vi "emballage nouvelle série_GPAO_OLD.vi"(1 "CodeBarFix":string, 2 "Nom du produit":string="12-216E-01-25 F120023 500mA 10Ohm", 3 "error in (no error)":errorcluster caption="entrée d'erreur (pas d'erreur)", 6 "Verif.Indice Client":bool) -> (5 "error out":errorcluster caption="sortie d'erreur", 11 "Indice Client":string, 14 "No commande FAS":string, 16 "DATA cmde":T1={"n°article FAS"="12-216E-01-25 F120023 500mA 10ohm", "n° cmde FAS"="R03844/08-01.01.01", "quantité cmde"="4", "ID LIG cmde"="225540", "n° cmde client"="120565              ", "nom client"="Fluid Automat. Systems GmbH", "n° article client"="21088", "indice revision client"="      ", "société de facturation"="FAS Medic SA                            ", "langue a utiliser"="ALL"}, 17 "Quantité de la commande":string="4", 18 "Commande interne":bool, 19 "Annuler(T=OK)":bool)   [LabVIEW 2020]
uses:
  VG_VerifTests_ModeRetour.vi
  Modules/FS/60_FS_Controles/60_FS_SetGet.ctl
panel:
  out "Cde_GPAO":bool
  in  "Cmde_Interne?":bool
  out "Indice Piece":string
  out "Tableau historique":string[][](array[string])=[["112105740008090004", "01.01.2001 01:01:00", "55", "01234/08-01.01.01", "1", "0"], ["112105740008090006", "01.01.2001 01:01:00", "55", "56789/08-01.01.01", "3", "0"], ["112105740008090007", "01.01.2001 01:01:00", "55", "56789/08-01.01.01", "4", "0"], ["112105740008090007", "01.01.2001 01:01:00", "55", "00123/08-01.01.01", "2", "1"]]
  out "Glissière 2":u8(slide)=100 caption="Identification terminé." scale=0.0..100.0
  in  "Valider qtté":bool
  in  "modifier qtté":bool
  in  "Numéro de commande FAS":string(combo)
  in  "Valider cmde":bool
  in  "Annuler?":bool
  # "La recherche se fait uniquement avec le numéro d'article et du numéro de file.\nLa designation (24V,...) n'est pas tenue compte (sauf pour les Flatprop) !!"
  # "Numéro de commande FAS"
  # "Seul un responsable peut valider une commande R (Retour)"
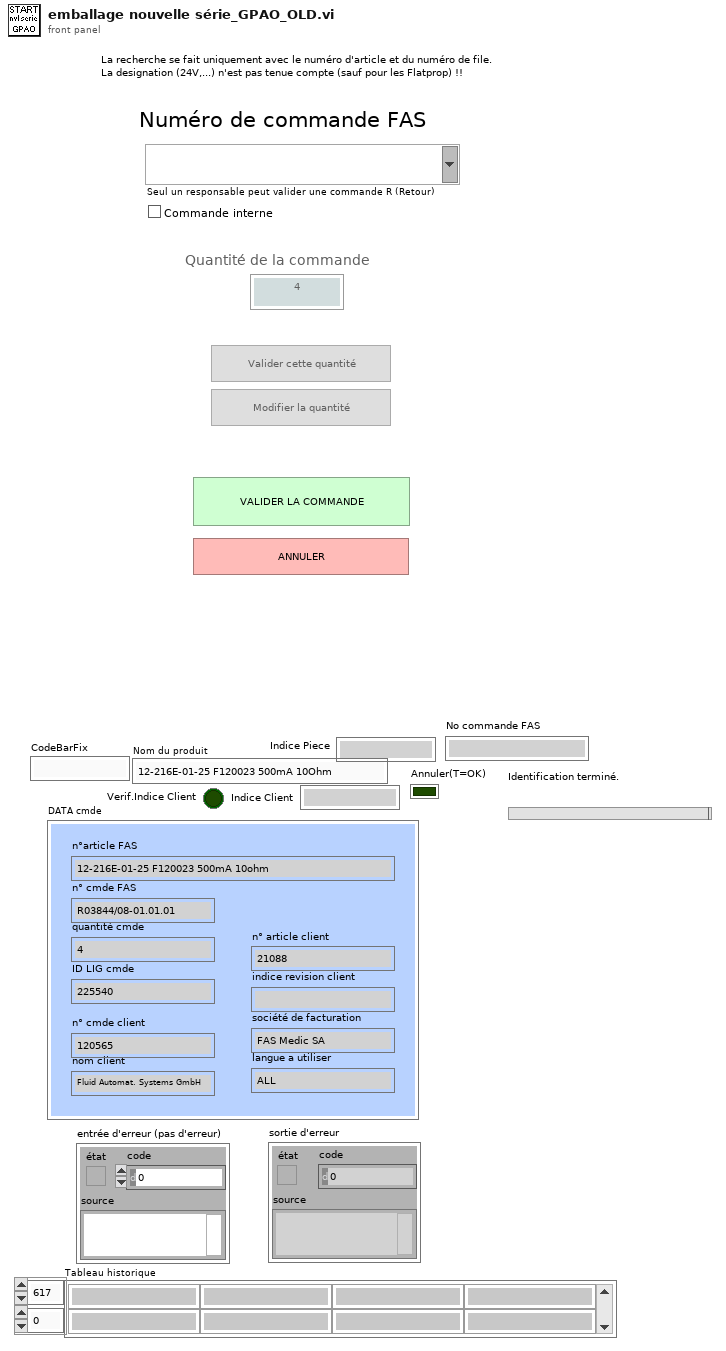
[diagram p1: front panel]
types:
  T1 = typedef "DATA commande.ctl" = cluster{"n°article FAS":string, "n° cmde FAS":string, "quantité cmde":string, "ID LIG cmde":string, "n° cmde client":string, "nom client":string, "n° article client":string, "indice revision client":string, "société de facturation":string, "langue a utiliser":string}
  T2 = typedef "60_FS_SetGet.ctl" = enum16{"set", "get"}
  T3 = enum16{"n° produit", "date", "opérateur", "n° cmde", "n° carton"}
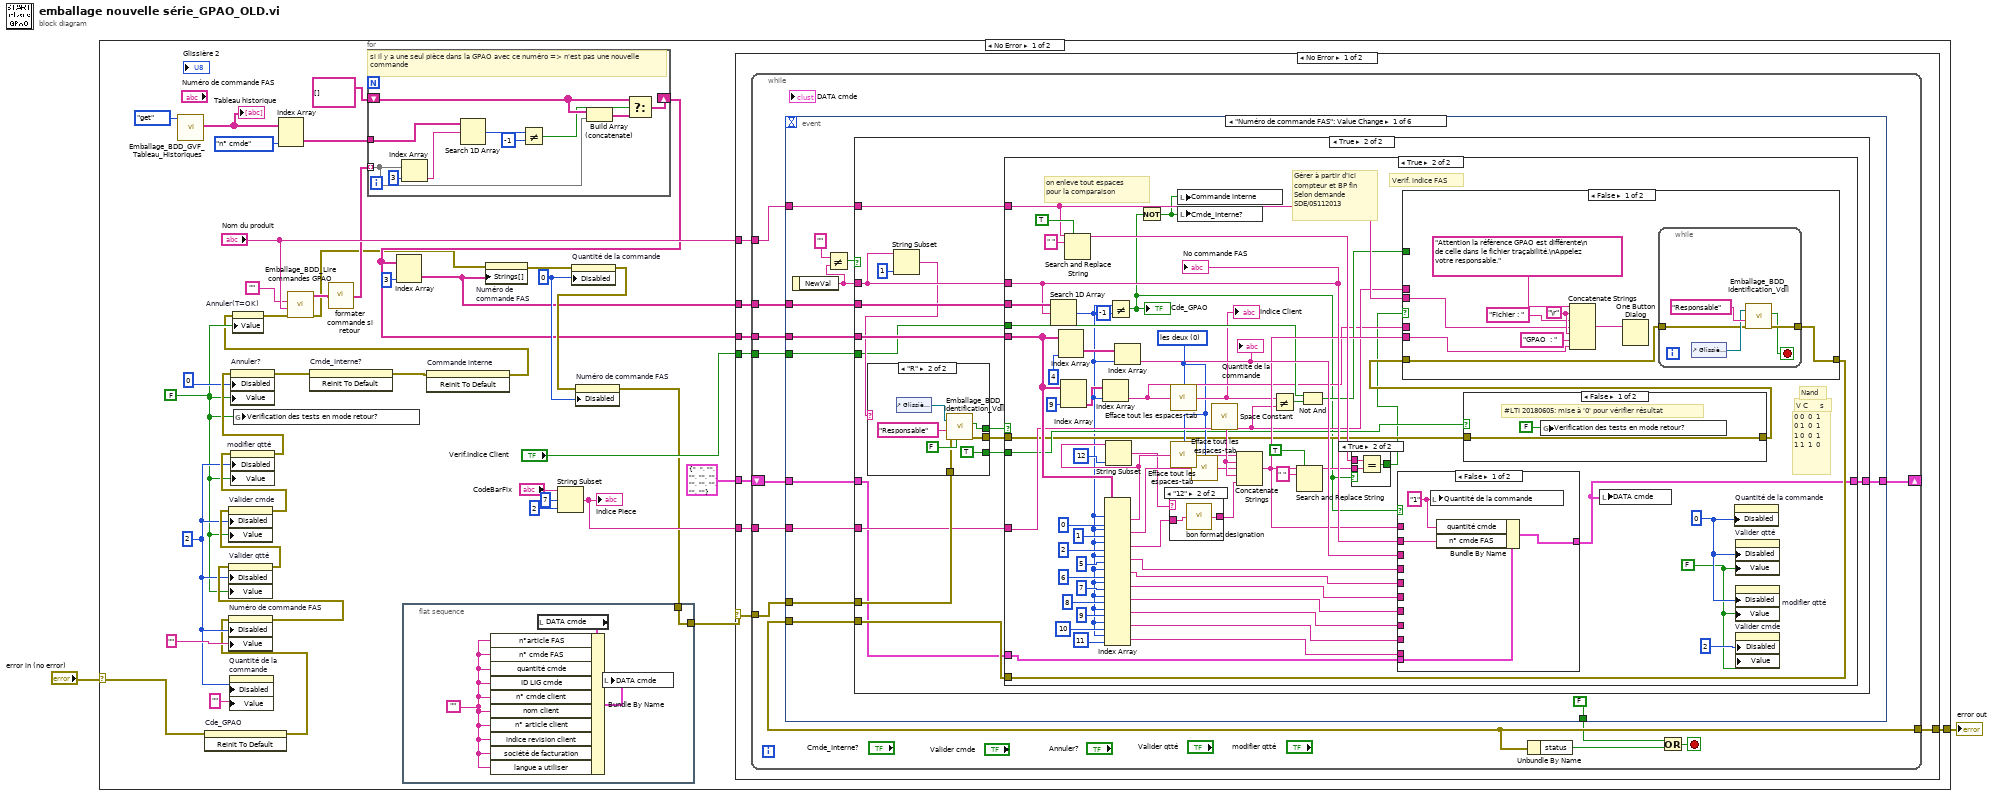
[diagram p0: block diagram]
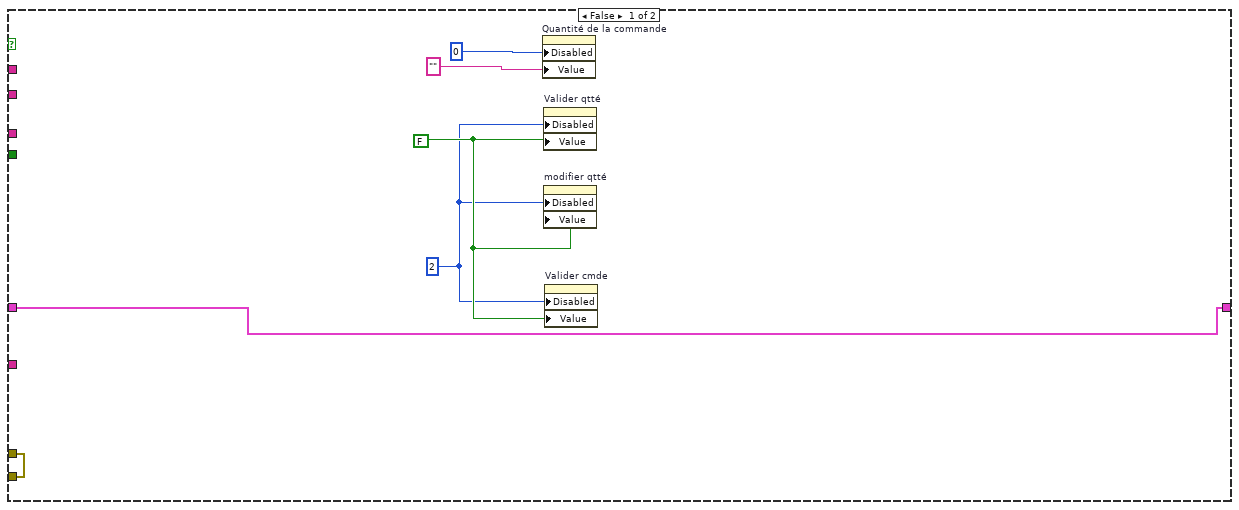
[diagram p2: hidden frame]
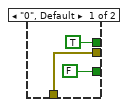
[diagram p3: hidden frame]
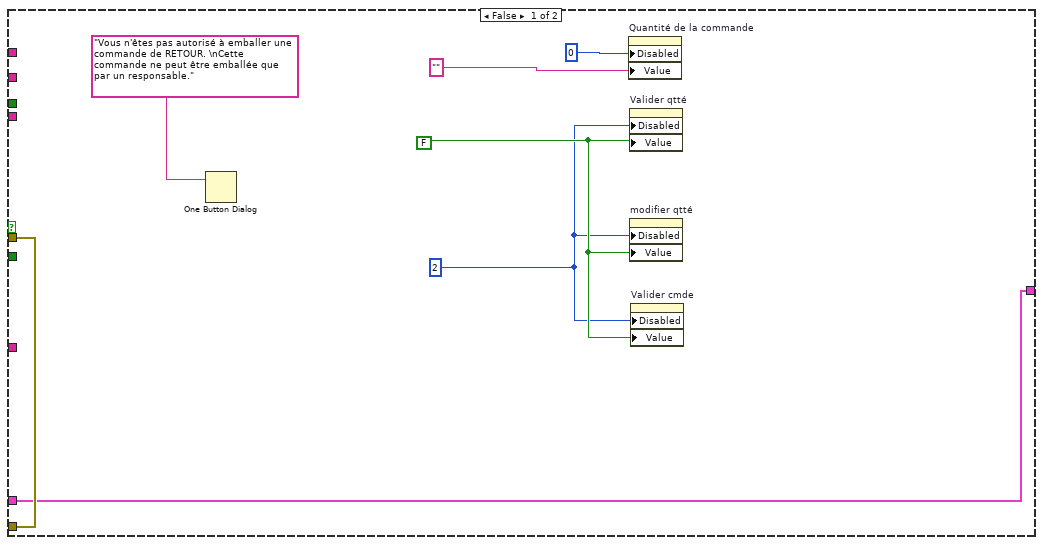
[diagram p4: hidden frame]
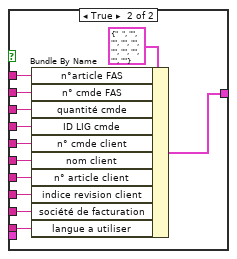
[diagram p5: hidden frame]
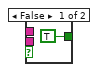
[diagram p6: hidden frame]
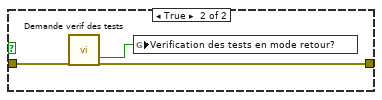
[diagram p7: hidden frame]
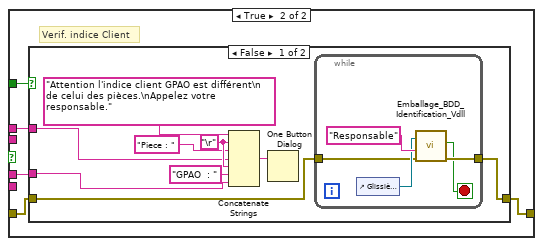
[diagram p8: hidden frame]
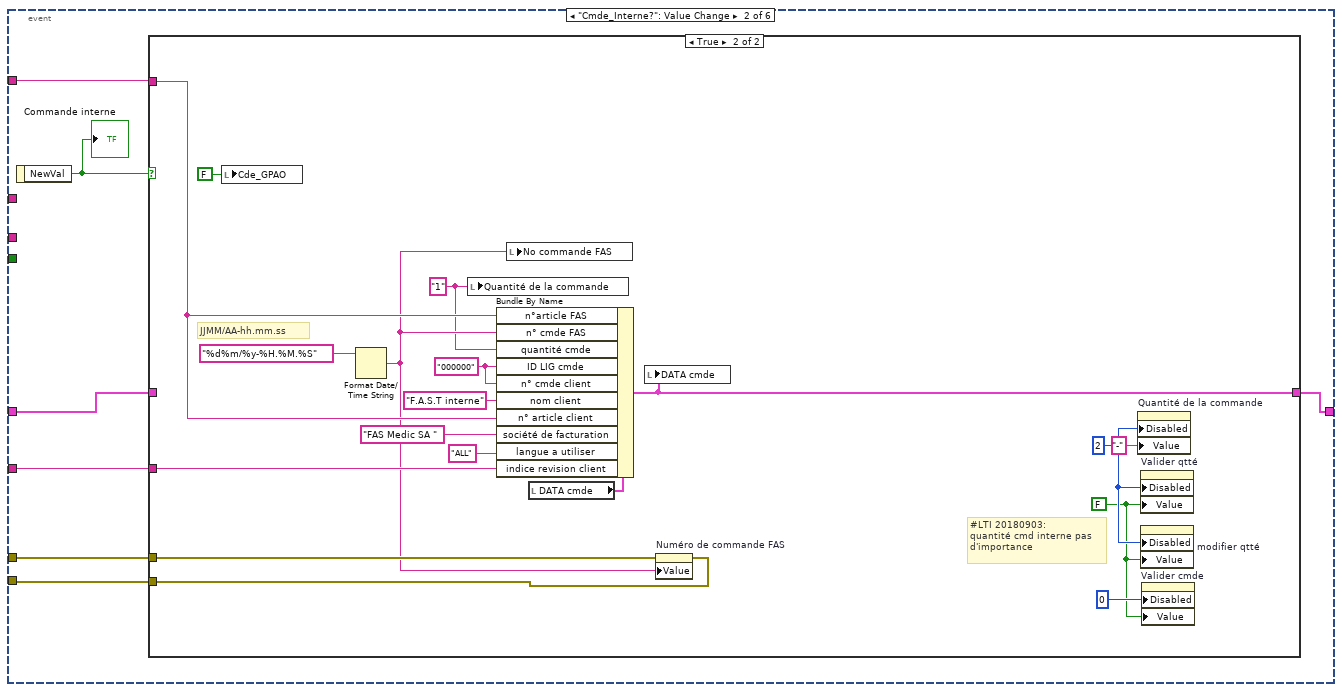
[diagram p11: hidden frame]
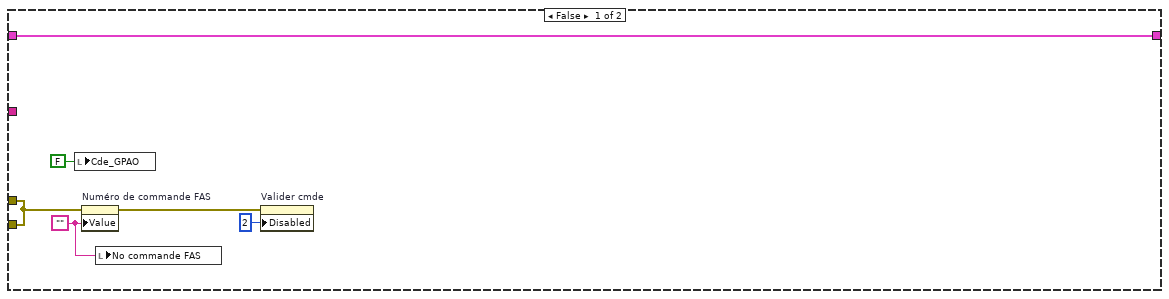
[diagram p12: hidden frame]
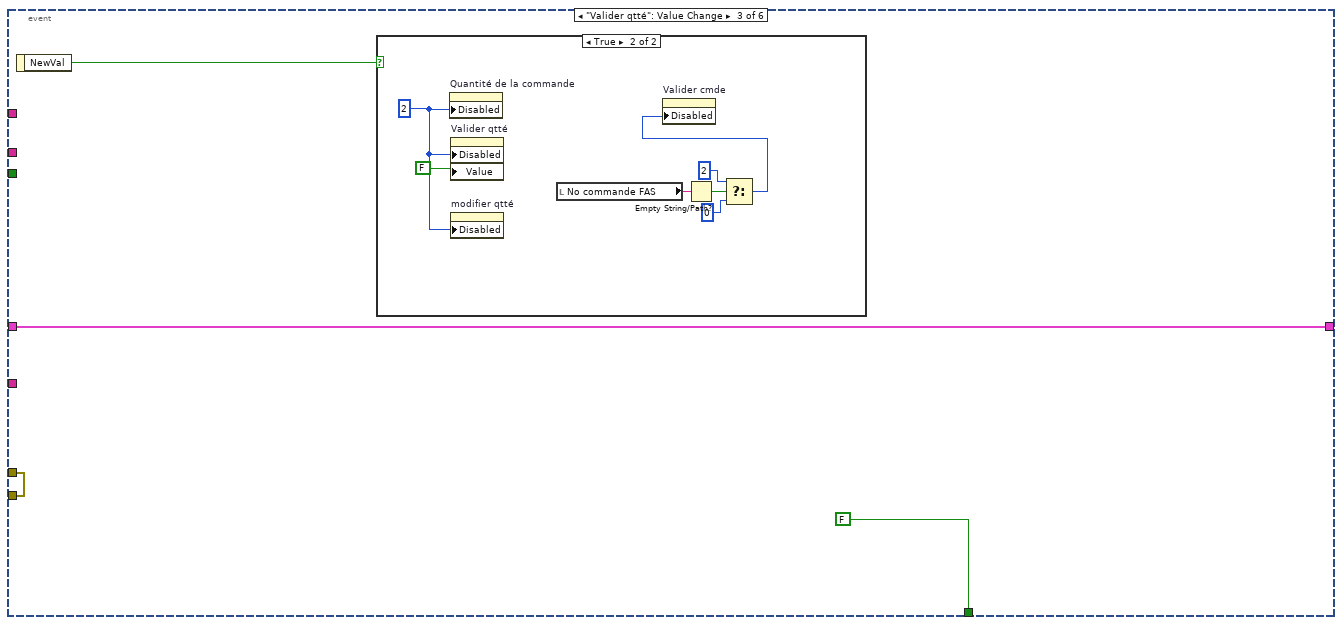
[diagram p13: hidden frame]
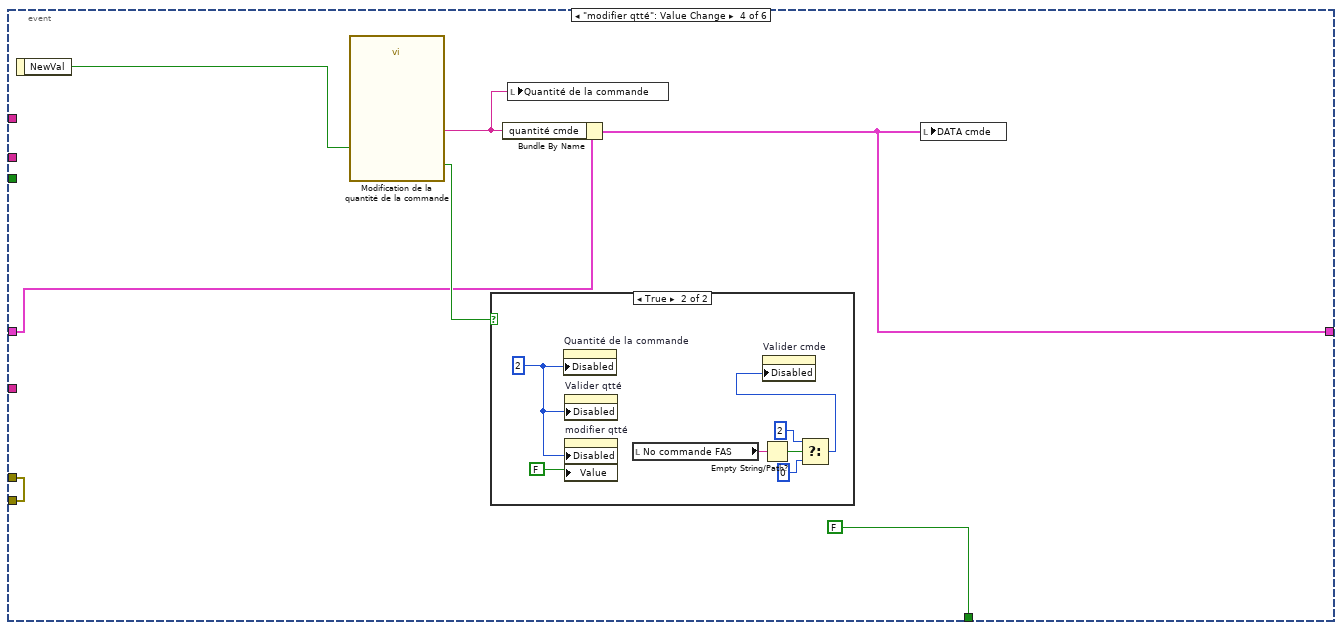
[diagram p15: hidden frame]
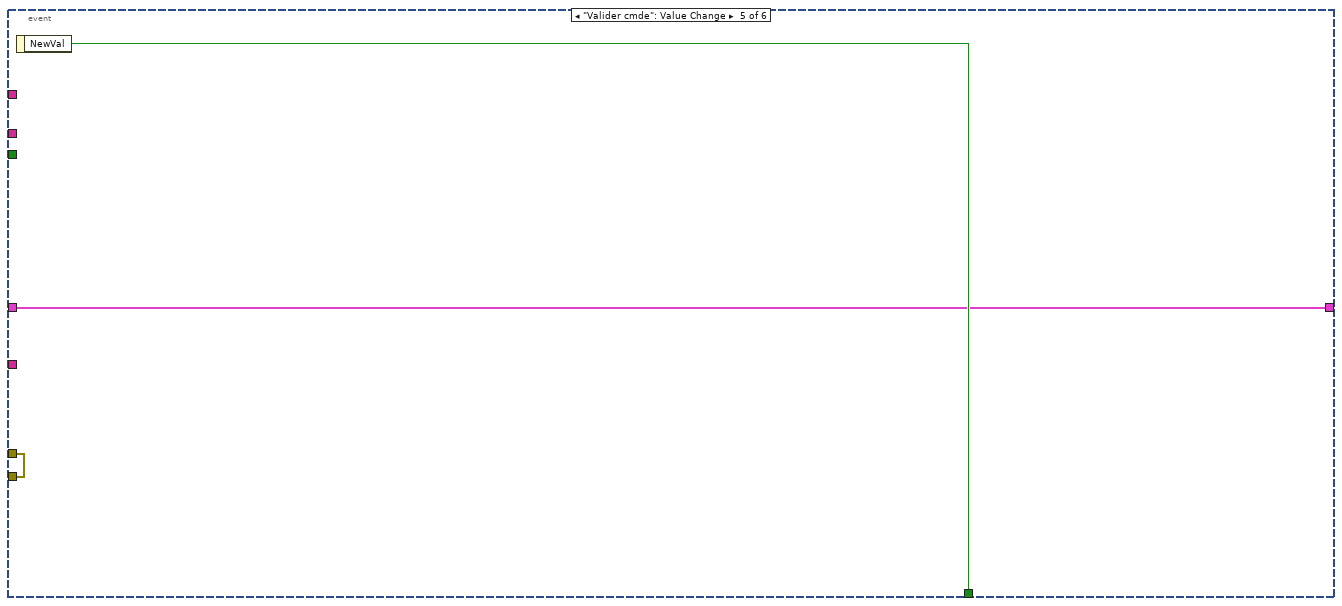
[diagram p17: hidden frame]
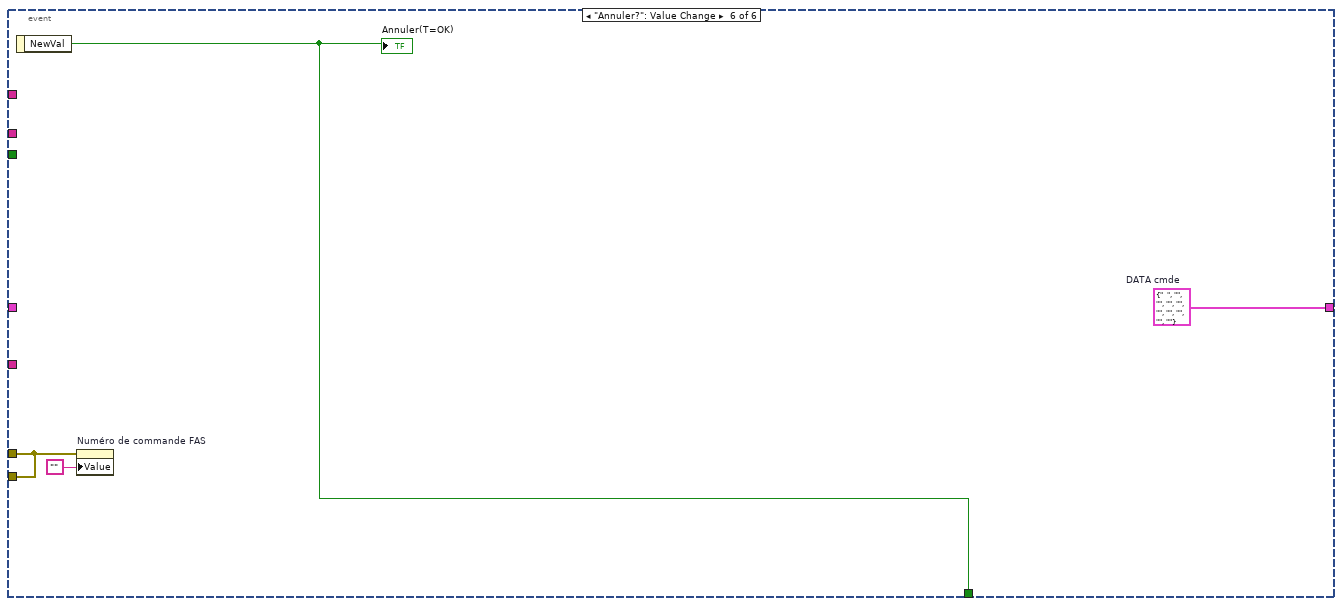
[diagram p18: hidden frame]
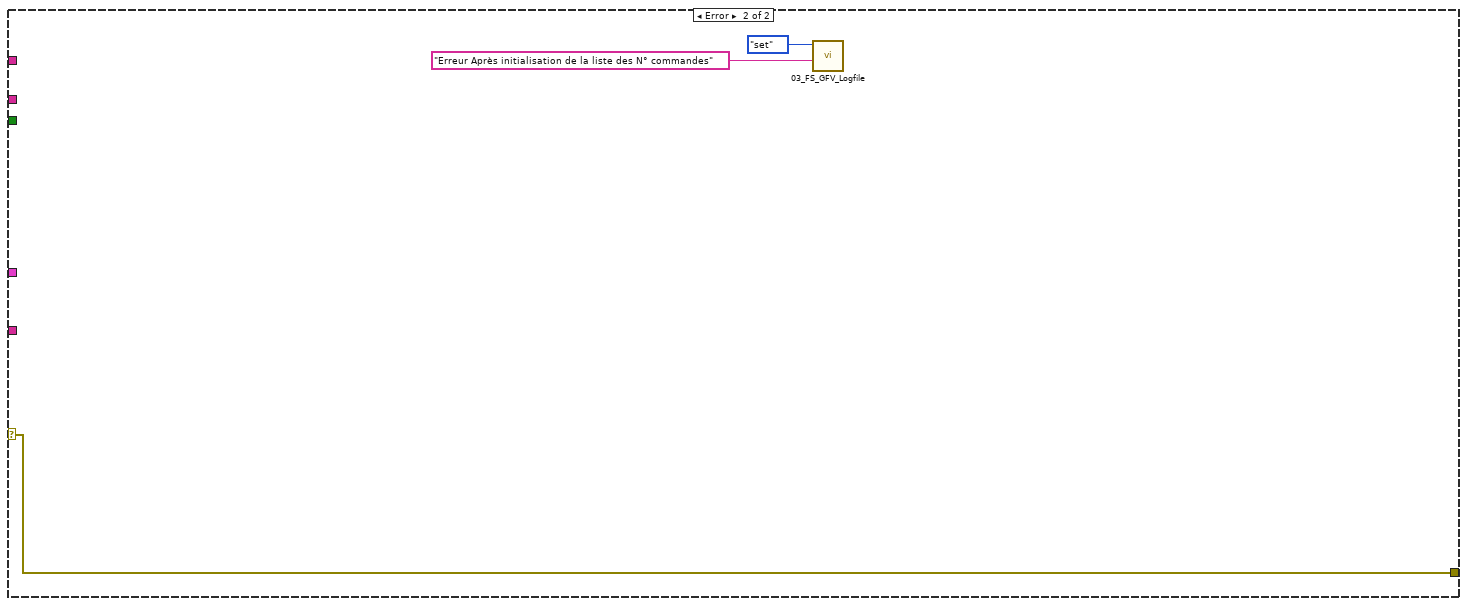
[diagram p19: hidden frame]
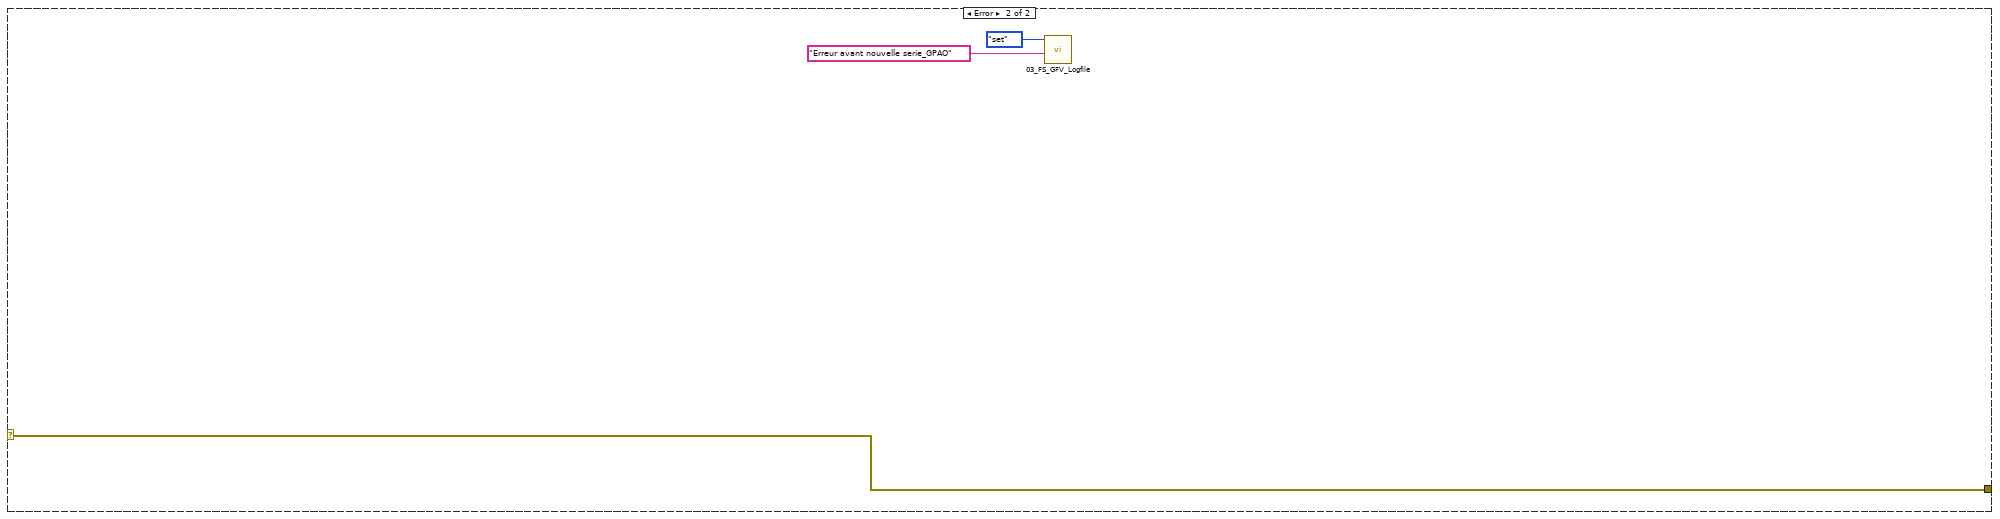
[diagram p20: hidden frame]
diagram:
  n1 = case shown="No Error" "error in (no error)" {
    selector: "error in (no error)" -> [w7 w321]
    tunnel: [w27 w321] -> w1
    frame No Error {
      w33 = u8 0 ("Désactivé")
      w37 = u8 2 ("Désactivé")
      w12 = FALSE
      n2 = call "Emballage_BDD_GVF_Tableau_Historiques.vi"("SetGet"=60_FS_SetGet."get") -> ("Tableau historique OUT"=w4:string[][])  [unwired: 9 in, 1 out]
      "Tableau historique" <- w4
      n3 = invoke on="Cde_GPAO" class="Bool (strict)" method="Reinit To Default"(error in=w7) -> (error out=w6:errorcluster)  [unwired: 2 in, 2 out]
      n4 = property on="Numéro de commande FAS" class="CmbBox"(error in=w6, "Disabled"=w37, "Value"="" ("Numéro de commande FAS")) -> (error out=w42:errorcluster)  [unwired: 1 in, 1 out]
      n5 = property on="Valider qtté" class="Bool (strict)"(error in=w42, "Disabled"=w37, "Value"=w12) -> (error out=w41:errorcluster)  [unwired: 1 in, 1 out]
      n6 = property on="Valider cmde" class="Bool (strict)"(error in=w41, "Disabled"=w37, "Value"=w12) -> (error out=w39:errorcluster)  [unwired: 1 in, 1 out]
      n7 = property on="Quantité de la commande" class="Str"("Disabled"=w37, "Value"="" ("Quantité de la commande")) -> ()  [unwired: 2 in, 2 out]
      n8 = property on="modifier qtté" class="Bool (strict)"(error in=w39, "Disabled"=w37, "Value"=w12) -> (error out=w38:errorcluster)  [unwired: 1 in, 1 out]
      n9 = property on="Annuler?" class="Bool (strict)"(error in=w38, "Disabled"=u8 0 ("Désactivé"), "Value"=w12) -> (error out=w11:errorcluster)  [unwired: 1 in, 1 out]
      n10 = global write "VG_VerifTests_ModeRetour.vi" "Verification des tests en mode retour?"(w12) -> ()
      n11 = Index Array(array=w4, index (col)=T3."n° cmde" ("Filtre")) -> (element=w24:string[])  [unwired: 1 in]
      n12 = invoke on="Cmde_Interne?" class="Bool (strict)" method="Reinit To Default"(error in=w11) -> (error out=w10:errorcluster)  [unwired: 2 in, 2 out]
      n13 = flat-sequence {
        tunnel: w8 -> [w316]
        tunnel: [w316] -> w28
        frame #0 {
          w315 = ""
          n14 = local read "DATA cmde"() -> (w318:T1)
          n15 = Bundle By Name(cluster=w318, "n°article FAS"=w315, "n° cmde FAS"=w315, "quantité cmde"=w315, "ID LIG cmde"=w315, "n° cmde client"=w315, "nom client"=w315, "n° article client"=w315, "indice revision client"=w315, "société de facturation"=w315, "langue a utiliser"=w315) -> (w317:T1)
          n16 = local write "DATA cmde"(w317) -> ()
        }
      }
      n17 = invoke on="Commande interne" class="Bool (strict)" method="Reinit To Default"(error in=w10) -> (error out=w9:errorcluster)  [unwired: 2 in, 2 out]
      n18 = property on="Annuler(T=OK)" class="Bool (strict)"(error in=w9, "Value"=w12) -> (error out=w31:errorcluster)  [unwired: 1 in, 1 out]
      n19 = call "Emballage_BDD_Lire  commandes GPAO.vi"("error in"=w31, "article"="Nom du produit", "Numéro commande"="") -> ("error out"=w19:errorcluster, "Tab cmde GPAO"=w29:string[][])  [unwired: 3 in, 4 out]
      n20 = call "formater commande si retour.vi"("Tab cmde GPAO IN"=w29) -> ("Tab cmde GPAO OUT"=w22:string[][])
      n21 = for {
        tunnel: w24 -> [w47]
        shift-right: [w52] -> w20
        shift-left: string[][] [] -> [w51]
        tunnel: w22 -> [w48] mode=indexing
        # "si il y a une seul pièce dans la GPAO avec ce numéro => n'est pas une nouvelle\ncommande"
        n22 = Index Array(array=w48, index=3 ("indice désactivé (col)")) -> (element=w46:string)
        n23 = Search 1D Array(1D array=w47, element=w46) -> (index of element=w45:i32)  [unwired: 1 in]
        n24 = Not Equal?(x=w45, y=-1) -> (x != y?=w43:bool)
        n25 = Build Array (concatenate)(w51, w48) -> (w50:string[][])
        n26 = Select(t=w51, s=w43, f=w50) -> (s? t:f=w52:string[][])
      }
      n27 = Index Array(array=w20, index (col)=3 ("indice désactivé (col)")) -> (element=w21:string[])  [unwired: 1 in]
      n28 = property on="Numéro de \ncommande FAS" class="CmbBox"(error in=w19, "Strings[]"=w21) -> (error out=w34:errorcluster)  [unwired: 1 in, 1 out]
      n29 = String Subset(string="CodeBarFix", offset (0)=7, length (rest)=2 ("longueur (reste)")) -> (substring=w14:string)
      "Indice Piece" <- w14
      n30 = property on="Quantité de la commande" class="Str"(error in=w34, "Disabled"=w33) -> (error out=w35:errorcluster)  [unwired: 1 in, 1 out]
      n31 = property on="Numéro de commande FAS" class="CmbBox"(error in=w35, "Disabled"=w33) -> (error out=w8:errorcluster)  [unwired: 1 in, 1 out]
      n32 = case shown="No Error" w28 {
        selector: w28 -> [w57 w314]
        tunnel: w21 -> [w60 _]
        tunnel: w20 -> [w59 _]
        tunnel: [w58 w314] -> w27
        tunnel: "Nom du produit" -> [w56 _]
        tunnel: w14 -> [w55 _]
        tunnel: "Verif.Indice Client" -> [w54 _]
        tunnel: T1 {"n°article FAS"="  ", "n° cmde FAS"="", "quantité cmde"="", "ID LIG cmde"="", "n° cmde client"="", "nom client"="", "n° article client"="", "indice revision client"="", "société de facturation"="", "langue a utiliser"=""} ("DATA cmde") -> [w53 _]
        frame No Error {
          n33 = while {
            tunnel: w60 -> [w72]
            tunnel: w59 -> [w71]
            tunnel: [w68] -> w58
            tunnel: w57 -> [w69]
            tunnel: w56 -> [w70]
            tunnel: w55 -> [w64]
            tunnel: w54 -> [w63]
            shift-right: [w62] -> _
            shift-left: w53 -> [w61]
            stop <- w67 stop-if-true
            n34 = event shown="[0] \"Numéro de commande FAS\": Value Change" {
              selector: _ -> [_ _ _ _ _ _]
              dyn-events: _ -> [_ _ _ _ _ _]
              timeout: _ -> [_ _ _ _ _ _]
              tunnel: w72 -> [w85 _ _ _ _ _]
              tunnel: w71 -> [w83 _ _ _ _ _]
              tunnel: [FALSE _ FALSE FALSE w307 w311] -> w66
              tunnel: w70 -> [w79 w252 _ _ _ _]
              tunnel: w69 -> [w78 w254 w281 w293 w306 w309]
              tunnel: [w77 w253 w281 w293 w306 w309] -> w68
              tunnel: w64 -> [w76 w251 _ _ _ _]
              tunnel: w63 -> [w75 _ _ _ _ _]
              tunnel: [w74 w250 w280 w291 w305 w308] -> w62
              tunnel: w61 -> [w73 w249 w280 w292 w305 _]
              event "Numéro de commande FAS": Value Change {
                n35 = event-data() -> ("NewVal"=w80:string)  [unwired: 1 in]
                n36 = Not Equal?(x="" ("nouvel élément/sous-tableau"), y=w80) -> (x != y?=w82:bool)
                n37 = case shown="True" w82 {
                  tunnel: w85 -> [_ w106]
                  tunnel: w80 -> [_ w104]
                  tunnel: w83 -> [_ w105]
                  tunnel: w79 -> [_ w100]
                  tunnel: w78 -> [w87 w99]
                  tunnel: [w87 w97] -> w77
                  tunnel: w76 -> [_ w96]
                  tunnel: w75 -> [_ w95]
                  tunnel: [w86 w93] -> w74
                  tunnel: w73 -> [w86 w92]
                  frame False {
                    w91 = FALSE
                    w88 = u8 2 ("Désactivé")
                    n38 = property on="Quantité de la commande" class="Str"("Disabled"=u8 0 ("Désactivé"), "Value"="" ("nouvel élément/sous-tableau")) -> ()  [unwired: 2 in, 2 out]
                    n39 = property on="Valider qtté" class="Bool (strict)"("Disabled"=w88, "Value"=w91) -> ()  [unwired: 2 in, 2 out]
                    n40 = property on="modifier qtté" class="Bool (strict)"("Disabled"=w88, "Value"=w91) -> ()  [unwired: 2 in, 2 out]
                    n41 = property on="Valider cmde" class="Bool (strict)"("Disabled"=w88, "Value"=w91) -> ()  [unwired: 2 in, 2 out]
                  }
                  frame True {
                    n42 = String Subset(string=w104, length (rest)=1 ("longueur (reste)")) -> (substring=w102:string)  [unwired: 1 in]
                    n43 = case shown="\"R\"" w102 {
                      tunnel: [TRUE w113] -> w101
                      tunnel: w99 -> [w108 w114]
                      tunnel: [w108 w111] -> w98
                      tunnel: [FALSE ("lecture seul possible ?") TRUE ("lecture seul possible ?")] -> w94
                      frame "0", Default {
                      }
                      frame "R" {
                        n44 = control-ref of="Glissière 2"() -> (w112:refnum<vi>)
                        n45 = call "Emballage_BDD_Identification_Vdll.vi"("Glissière"=w112, "lecture seul possible ?"=FALSE, "error in"=w114, "Posage choisi"="Responsable") -> ("error Out"=w111:errorcluster, "OK"=w113:bool)  [unwired: 3 in, 3 out]
                      }
                    }
                    n46 = case shown="True" w101 {
                      tunnel: w106 -> [_ w186]
                      tunnel: w104 -> [_ w178]
                      tunnel: w105 -> [_ w143]
                      tunnel: w100 -> [_ w145]
                      tunnel: w98 -> [w118 w131]
                      tunnel: [w118 w144] -> w97
                      tunnel: w96 -> [_ w138]
                      tunnel: w95 -> [_ w137]
                      tunnel: w94 -> [_ w132]
                      tunnel: [w117 w126] -> w93
                      tunnel: w92 -> [w117 w125]
                      frame False {
                        w122 = FALSE
                        w119 = u8 2 ("Désactivé")
                        n47 = One Button Dialog(message="Vous n'êtes pas autorisé à emballer une commande de RETOUR. \nCette commande ne peut être emballée que par un responsable.") -> ()  [unwired: 1 in, 1 out]
                        n48 = property on="Quantité de la commande" class="Str"("Disabled"=u8 0 ("Désactivé"), "Value"="" ("nouvel élément/sous-tableau")) -> ()  [unwired: 2 in, 2 out]
                        n49 = property on="Valider qtté" class="Bool (strict)"("Disabled"=w119, "Value"=w122) -> ()  [unwired: 2 in, 2 out]
                        n50 = property on="modifier qtté" class="Bool (strict)"("Disabled"=w119, "Value"=w122) -> ()  [unwired: 2 in, 2 out]
                        n51 = property on="Valider cmde" class="Bool (strict)"("Disabled"=w119, "Value"=w122) -> ()  [unwired: 2 in, 2 out]
                      }
                      frame True {
                        w134 = u16 0 items=["les deux", "début de la chaîne", "fin de chaîne"] ("location (both)")
                        w170 = FALSE
                        w174 = u8 0 ("Désactivé")
                        # "Gérer à partir d'ici \ncompteur et BP fin\nSelon demande \nSDE/05112013"
                        # "Nand"
                        # "V C      s"
                        # "0 0  0  1\n0 1  0  1\n1 0  0  1\n1 1  1  0"
                        # "Verif. indice FAS"
                        # "on enleve tout espaces \npour la comparaison"
                        n52 = Search 1D Array(1D array=w186, element=w178) -> (index of element=w129:i32)  [unwired: 1 in]
                        n53 = Index Array(array=w143, index (col)=4 ("indice désactivé (col)")) -> (element=w171:string[])  [unwired: 1 in]
                        n54 = Index Array(array=w143, index (col)=9 ("indice désactivé (col)")) -> (element=w141:string[])  [unwired: 1 in]
                        n55 = Search and Replace String(replace all?=TRUE ("tout remplacer ? (F)"), input string=w145, search string=" " ("chaîne recherchée")) -> (result string=w151:string)  [unwired: 5 in, 3 out]
                        n56 = Index Array(array=w141, index=w129) -> (element=w136:string)
                        n57 = Index Array(array=w143, index (row) #1=w129, index (col) #1=0 ("indice désactivé (col)"), index (row) #2=w129, index (col) #2=1 ("indice désactivé (col)"), index (row) #3=w129, index (col) #3=2 ("indice désactivé (col)"), index (row) #4=w129, index (col) #4=5 ("indice désactivé (col)"), index (row) #5=w129, index (col) #5=6 ("indice désactivé (col)"), index (row) #6=w129, index (col) #6=7 ("indice désactivé (col)"), index (row) #7=w129, index (col) #7=8 ("indice désactivé (col)"), index (row) #8=w129, index (col) #8=9 ("indice désactivé (col)"), index (row) #9=w129, index (col) #9=10 ("indice désactivé (col)"), index (row) #10=w129, index (col) #10=11 ("indice désactivé (col)")) -> (element #1=w156:string, element #2=w164:string, element #3=w153:string, element #4=w176:string, element #5=w175:string, element #6=w162:string, element #7=w161:string, element #8=w160:string, element #9=w159:string, element #10=w158:string)
                        n58 = String Subset(string=w156, length (rest)=12 ("longueur (reste)")) -> (substring=w154:string)  [unwired: 1 in]
                        n59 = Not Equal?(x=w129, y=-1) -> (x != y?=w124:bool)
                        "Cde_GPAO" <- w124
                        n60 = Index Array(array=w171, index=w129) -> (element=w177:string)
                        "Quantité de la commande" <- w177
                        n61 = Not(x=w124) -> (.not. x?=w127:bool)
                        n62 = case shown="\"12\"" w154 {
                          tunnel: [w246 w248] -> w157
                          tunnel: w153 -> [w246 w247]
                          frame Default {
                          }
                          frame "12" {
                            n63 = call "bon format designation.vi"("Chaîne IN"=w247) -> ("Chaîne OUT"=w248:string)
                          }
                        }
                        n64 = call "Efface tout les espaces-tab.vi"("string"=w136, "location (both)"=w134) -> ("trimmed string"=w135:string)
                        "Indice Client" <- w135
                        n65 = call "Efface tout les espaces-tab.vi"("string"=w156, "location (both)"=w134) -> ("trimmed string"=w165:string)
                        n66 = local write "Commande interne"(w127) -> ()
                        n67 = local write "Cmde_Interne?"(w127) -> ()
                        n68 = call "Efface tout les espaces-tab.vi"("string"=w164, "location (both)"=w134) -> ("trimmed string"=w163:string)
                        n69 = call <vilib>:"Space Constant.vi"() -> ("String"=w166:string)
                        n70 = Concatenate Strings(w165, w166, w163, w166, w157) -> (w146:string)
                        n71 = Not Equal?(x=w135, y=w138) -> (x != y?=w140:bool)
                        n72 = Search and Replace String(replace all?=TRUE ("tout remplacer ? (F)"), input string=w146, search string=" " ("chaîne recherchée")) -> (result string=w148:string)  [unwired: 5 in, 3 out]
                        n73 = Not And(1:w140, 2:w137) -> (0:w139:bool)
                        n74 = case shown="True" w124 {
                          tunnel: w151 -> [_ w206]
                          tunnel: w148 -> [_ w205]
                          tunnel: [TRUE w204] -> w130
                          frame False {
                          }
                          frame True {
                            n75 = Equal?(x=w206, y=w205) -> (x = y?=w204:bool)
                          }
                        }
                        n76 = case shown="False" w124 {
                          tunnel: w178 -> [w190 w202]
                          tunnel: w177 -> [_ w201]
                          tunnel: w176 -> [_ w200]
                          tunnel: w175 -> [_ w199]
                          tunnel: w162 -> [_ w198]
                          tunnel: w161 -> [_ w197]
                          tunnel: w160 -> [_ w196]
                          tunnel: w159 -> [_ w195]
                          tunnel: w158 -> [_ w194]
                          tunnel: w146 -> [_ w193]
                          tunnel: [w188 w191] -> w126
                          tunnel: w125 -> [w189 _]
                          frame False {
                            w187 = "1" ("Quantité de la commande")
                            n77 = local write "Quantité de la commande"(w187) -> ()
                            n78 = Bundle By Name(cluster=w189, "quantité cmde"=w187, "n° cmde FAS"=w190) -> (w188:T1)
                          }
                          frame True {
                            n79 = Bundle By Name(cluster=T1 {"n°article FAS"="  ", "n° cmde FAS"="", "quantité cmde"="", "ID LIG cmde"="", "n° cmde client"="", "nom client"="", "n° article client"="", "indice revision client"="", "société de facturation"="", "langue a utiliser"=""} ("DATA cmde"), "n°article FAS"=w193, "n° cmde FAS"=w202, "quantité cmde"=w201, "ID LIG cmde"=w200, "n° cmde client"=w199, "nom client"=w198, "n° article client"=w197, "indice revision client"=w196, "société de facturation"=w195, "langue a utiliser"=w194) -> (w191:T1)
                          }
                        }
                        n80 = case shown="False" w132 {
                          tunnel: w131 -> [w208 w211]
                          tunnel: [w208 w210] -> w133
                          frame False {
                            # "#LTI 20180605: mise à '0' pour vérifier résultat"
                            n81 = global write "VG_VerifTests_ModeRetour.vi" "Verification des tests en mode retour?"(FALSE ("Verification des tests en mode retour?")) -> ()
                          }
                          frame True {
                            n82 = call "Demande verif des tests"("error in (no error)"=w211) -> ("OUI"=w209:bool, "error out"=w210:errorcluster)  [unwired: 17 in]
                            n83 = global write "VG_VerifTests_ModeRetour.vi" "Verification des tests en mode retour?"(w209) -> ()
                          }
                        }
                        n84 = case shown="False" w130 {
                          tunnel: w145 -> [w217 _]
                          tunnel: w146 -> [w215 _]
                          tunnel: w133 -> [w213 w230]
                          tunnel: [w212 w229] -> w144
                          tunnel: w136 -> [_ w228]
                          tunnel: w138 -> [_ w227]
                          tunnel: w139 -> [_ w226]
                          frame False {
                            w218 = "\r"
                            n85 = Concatenate Strings("Attention la référence GPAO est différente\n de celle dans le fichier traçabilité.\nAppelez votre responsable." ("message"), w218, "Fichier : " ("chaîne"), w217, w218, "GPAO  : " ("chaîne"), w215) -> (w220:string)
                            n86 = One Button Dialog(message=w220) -> ()  [unwired: 1 in, 1 out]
                            n87 = while {
                              tunnel: w213 -> [w223]
                              tunnel: [w222] -> w212
                              stop <- w221 stop-if-true
                              n88 = control-ref of="Glissière 2"() -> (w224:refnum<vi>)
                              n89 = call "Emballage_BDD_Identification_Vdll.vi"("Glissière"=w224, "error in"=w223, "Posage choisi"="Responsable") -> ("error Out"=w222:errorcluster, "OK"=w221:bool)  [unwired: 4 in, 3 out]
                            }
                          }
                          frame True {
                            # "Verif. indice Client"
                            n90 = case shown="False" w226 {
                              tunnel: w227 -> [w236 _]
                              tunnel: w228 -> [w234 _]
                              tunnel: w230 -> [w232 w245]
                              tunnel: [w231 w245] -> w229
                              frame False {
                                w237 = "\r"
                                n91 = Concatenate Strings("Attention l'indice client GPAO est différent\n de celui des pièces.\nAppelez votre responsable." ("message"), w237, "Piece : " ("chaîne"), w236, w237, "GPAO  : " ("chaîne"), w234) -> (w239:string)
                                n92 = One Button Dialog(message=w239) -> ()  [unwired: 1 in, 1 out]
                                n93 = while {
                                tunnel: w232 -> [w242]
                                tunnel: [w241] -> w231
                                stop <- w240 stop-if-true
                                n94 = control-ref of="Glissière 2"() -> (w243:refnum<vi>)
                                n95 = call "Emballage_BDD_Identification_Vdll.vi"("Glissière"=w243, "error in"=w242, "Posage choisi"="Responsable") -> ("error Out"=w241:errorcluster, "OK"=w240:bool)  [unwired: 4 in, 3 out]
                                }
                              }
                              frame True {
                                # "pas de vérifs ou indices OK"
                              }
                            }
                          }
                        }
                        n96 = local write "DATA cmde"(w126) -> ()
                        n97 = property on="Quantité de la commande" class="Str"("Disabled"=w174) -> ()  [unwired: 2 in, 2 out]
                        n98 = property on="Valider qtté" class="Bool (strict)"("Disabled"=w174, "Value"=w170) -> ()  [unwired: 2 in, 2 out]
                        n99 = property on="modifier qtté" class="Bool (strict)"("Disabled"=w174, "Value"=w170) -> ()  [unwired: 2 in, 2 out]
                        n100 = property on="Valider cmde" class="Bool (strict)"("Disabled"=u8 2 ("Désactivé"), "Value"=w170) -> ()  [unwired: 2 in, 2 out]
                        "No commande FAS" <- w178
                      }
                    }
                  }
                }
              }
              event "Cmde_Interne?": Value Change {
                n101 = event-data() -> ("NewVal"=w255:bool)  [unwired: 1 in]
                "Commande interne" <- w255
                n102 = case shown="True" w255 {
                  tunnel: w254 -> [w261 w269]
                  tunnel: [w261 w268] -> w253
                  tunnel: w252 -> [_ w273]
                  tunnel: w251 -> [_ w270]
                  tunnel: [w258 w264] -> w250
                  tunnel: w249 -> [w258 _]
                  frame False {
                    w260 = ""
                    n103 = local write "Cde_GPAO"(FALSE ("Cde_GPAO")) -> ()
                    n104 = property on="Numéro de commande FAS" class="CmbBox"(error in=w261, "Value"=w260) -> (error out=w256:errorcluster)  [unwired: 1 in, 1 out]
                    n105 = local write "No commande FAS"(w260) -> ()
                    n106 = property on="Valider cmde" class="Bool (strict)"(error in=w256, "Disabled"=u8 2 ("Désactivé")) -> ()  [unwired: 1 in, 2 out]
                  }
                  frame True {
                    w263 = "1" ("Quantité de la commande")
                    w275 = "000000" ("ID LIG cmde")
                    w276 = FALSE
                    w278 = u8 2 ("Désactivé")
                    # "#LTI 20180903:\nquantité cmd interne pas \nd'importance"
                    # "JJMM/AA-hh.mm.ss"
                    n107 = local write "Cde_GPAO"(FALSE ("Cde_GPAO")) -> ()
                    n108 = Format Date/Time String(time format string (%c)="%d%m/%y-%H.%M.%S" ("chaîne de format de l'heure (%c)")) -> (date/time string=w266:string)  [unwired: 2 in]
                    n109 = local write "Quantité de la commande"(w263) -> ()
                    n110 = local write "No commande FAS"(w266) -> ()
                    n111 = local read "DATA cmde"() -> (w279:T1)
                    n112 = Bundle By Name(cluster=w279, "n°article FAS"=w273, "n° cmde FAS"=w266, "quantité cmde"=w263, "ID LIG cmde"=w275, "n° cmde client"=w275, "nom client"="F.A.S.T interne", "n° article client"=w273, "société de facturation"="FAS Medic SA ", "langue a utiliser"="ALL", "indice revision client"=w270) -> (w264:T1)
                    n113 = local write "DATA cmde"(w264) -> ()
                    n114 = property on="Numéro de commande FAS" class="CmbBox"(error in=w269, "Value"=w266) -> (error out=w268:errorcluster)  [unwired: 1 in, 1 out]
                    n115 = property on="Quantité de la commande" class="Str"("Disabled"=w278, "Value"="-" ("Quantité de la commande")) -> ()  [unwired: 2 in, 2 out]
                    n116 = property on="Valider qtté" class="Bool (strict)"("Disabled"=w278, "Value"=w276) -> ()  [unwired: 2 in, 2 out]
                    n117 = property on="modifier qtté" class="Bool (strict)"("Disabled"=w278, "Value"=w276) -> ()  [unwired: 2 in, 2 out]
                    n118 = property on="Valider cmde" class="Bool (strict)"("Disabled"=u8 0 ("Désactivé"), "Value"=w276) -> ()  [unwired: 2 in, 2 out]
                  }
                }
              }
              event "Valider qtté": Value Change {
                n119 = event-data() -> ("NewVal"=w283:bool)  [unwired: 1 in]
                n120 = case shown="True" w283 {
                  frame False {
                  }
                  frame True {
                    w290 = u8 2 ("Désactivé")
                    n121 = property on="Quantité de la commande" class="Str"("Disabled"=w290) -> ()  [unwired: 2 in, 2 out]
                    n122 = property on="Valider qtté" class="Bool (strict)"("Disabled"=w290, "Value"=FALSE ("Valider qtté")) -> ()  [unwired: 2 in, 2 out]
                    n123 = property on="modifier qtté" class="Bool (strict)"("Disabled"=w290) -> ()  [unwired: 2 in, 2 out]
                    n124 = local read "No commande FAS"() -> (w288:string)
                    n125 = Empty String/Path?(string/path=w288) -> (empty?=w287:bool)
                    n126 = Select(t=u8 2 ("Désactivé"), s=w287, f=u8 0 ("Désactivé")) -> (s? t:f=w284:u8)
                    n127 = property on="Valider cmde" class="Bool (strict)"("Disabled"=w284) -> ()  [unwired: 2 in, 2 out]
                  }
                }
              }
              event "modifier qtté": Value Change {
                n128 = event-data() -> ("NewVal"=w295:bool)  [unwired: 1 in]
                n129 = call "Modification de la quantité de la commande"("Enable"=w295) -> ("Nouvelle quantité :"=w296:string, "OK"=w294:bool)  [unwired: 16 in, 1 out]
                n130 = case shown="True" w294 {
                  frame False {
                  }
                  frame True {
                    w304 = u8 2 ("Désactivé")
                    n131 = property on="Quantité de la commande" class="Str"("Disabled"=w304) -> ()  [unwired: 2 in, 2 out]
                    n132 = property on="Valider qtté" class="Bool (strict)"("Disabled"=w304) -> ()  [unwired: 2 in, 2 out]
                    n133 = property on="modifier qtté" class="Bool (strict)"("Disabled"=w304, "Value"=FALSE ("modifier qtté")) -> ()  [unwired: 2 in, 2 out]
                    n134 = local read "No commande FAS"() -> (w302:string)
                    n135 = Empty String/Path?(string/path=w302) -> (empty?=w301:bool)
                    n136 = Select(t=u8 2 ("Désactivé"), s=w301, f=u8 0 ("Désactivé")) -> (s? t:f=w298:u8)
                    n137 = property on="Valider cmde" class="Bool (strict)"("Disabled"=w298) -> ()  [unwired: 2 in, 2 out]
                  }
                }
                n138 = Bundle By Name(cluster=w292, "quantité cmde"=w296) -> (w291:T1)
                n139 = local write "Quantité de la commande"(w296) -> ()
                n140 = local write "DATA cmde"(w291) -> ()
              }
              event "Valider cmde": Value Change {
                n141 = event-data() -> ("NewVal"=w307:bool)  [unwired: 1 in]
              }
              event "Annuler?": Value Change {
                w308 = T1 {"n°article FAS"="  ", "n° cmde FAS"="", "quantité cmde"="", "ID LIG cmde"="", "n° cmde client"="", "nom client"="", "n° article client"="", "indice revision client"="", "société de facturation"="", "langue a utiliser"=""}  # DATA cmde
                n142 = event-data() -> ("NewVal"=w311:bool)  [unwired: 1 in]
                "Annuler(T=OK)" <- w311
                n143 = property on="Numéro de commande FAS" class="CmbBox"(error in=w309, "Value"="") -> ()  [unwired: 1 in, 2 out]
              }
            }
            n144 = Unbundle By Name(w68) -> ("status"=w65:bool)
            n145 = Or(x=w66, y=w65) -> (x .or. y?=w67:bool)
          }
        }
        frame Error {
          n146 = call "03_FS_GFV_Logfile.vi"("Chaîne"="Erreur Après initialisation de la liste des N° commandes", "States"=60_FS_SetGet."set") -> ()  [unwired: 8 in, 2 out]
        }
      }
    }
    frame Error {
      n147 = call "03_FS_GFV_Logfile.vi"("Chaîne"="Erreur avant nouvelle serie_GPAO", "States"=60_FS_SetGet."set") -> ()  [unwired: 8 in, 2 out]
    }
  }
  "error out" <- w1
